vi "PyLoN_data_recoveryTRYFIX.vi"(0 "Camera Handle":u32, 1 "Number of Images":u32=1 min=1 step=1, 5 "PumpOnBkgd":dbl[](array[numeric]), 7 "refnum":refnum<file>, 9 "PumpOffBkgd":dbl[](array[numeric]), 11 "error in (no error)":errorcluster) -> (3 "x/y":dbl, 4 "Camera Handle 2":u32 caption="Camera Handle", 6 "Pump_On":dbl[](array[numeric]), 8 "refnum out":refnum<file>, 10 "Pump_Off":dbl[](array[numeric]), 12 "Raman Data":dbl[][](array[numeric]), 13 "x > y?":bool, 14 "Raman_Gain":dbl[](array[numeric]), 15 "error out":errorcluster)   [LabVIEW 2015]
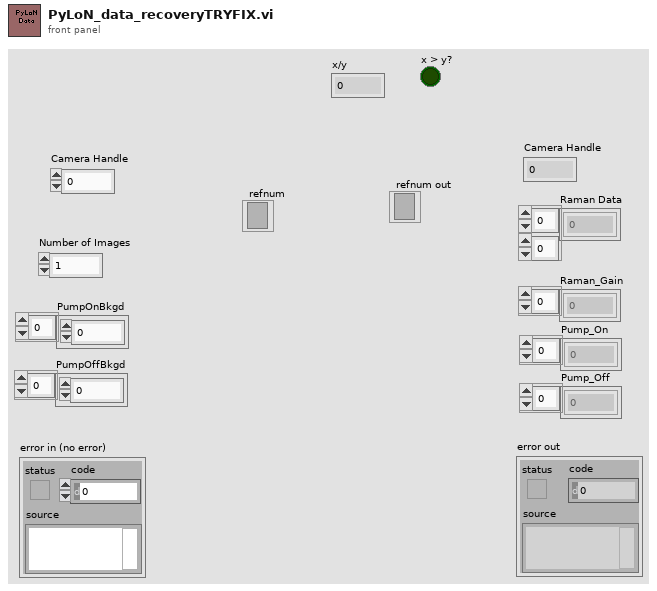
[diagram p1: front panel]
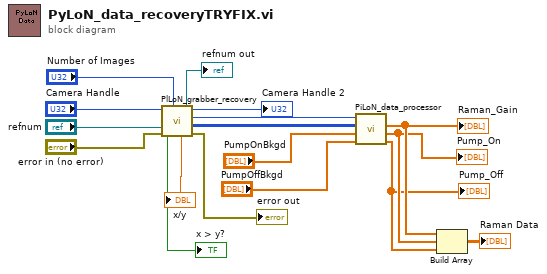
[diagram p0: block diagram]
diagram:
  n1 = call "PlLoN_grabber_recovery.vi"("Number of Images"="Number of Images", "error in (no error)"="error in (no error)", "refnum"="refnum", "Camera Handle"="Camera Handle") -> ("error out"=→"error out":errorcluster, "DATA"=w16:u16[][], "Number of Images"=w17:u32, "Camera Handle"=→"Camera Handle 2":u32, "x/y"=→"x/y":dbl, "refnum out"=→"refnum out":refnum<file>, "x > y?"=→"x > y?":bool)  [unwired: 1 in]
  n2 = call "PiLoN_data_processor.vi"("PumpOffBkgd"="PumpOffBkgd", "PumpOnBkgd"="PumpOnBkgd", "Data"=w16, "# of Images"=w17) -> ("Pump_Off"=w5:dbl[], "Pump_On"=w6:dbl[], "Raman_Gain"=w7:dbl[])  [unwired: 5 in]
  "Raman_Gain" <- w7
  "Pump_On" <- w6
  "Pump_Off" <- w5
  n3 = Build Array(w7, w6, w5) -> (→"Raman Data":dbl[][])
